vi "Analysis.Result Summaries, Generate Yield Per Day_V3.vi"(8 "LP Yield":dbl[](array[numeric]), 10 "FP Yield":dbl[](array[numeric]), 11 "Dates":timestamp[](array[timestamp])) -> (2 "Yield Per Date":string[][](table), 3 "Yield vs Date":cluster{"Dates":timestamp[], dbl[]}[](graph))   [LabVIEW 2024]
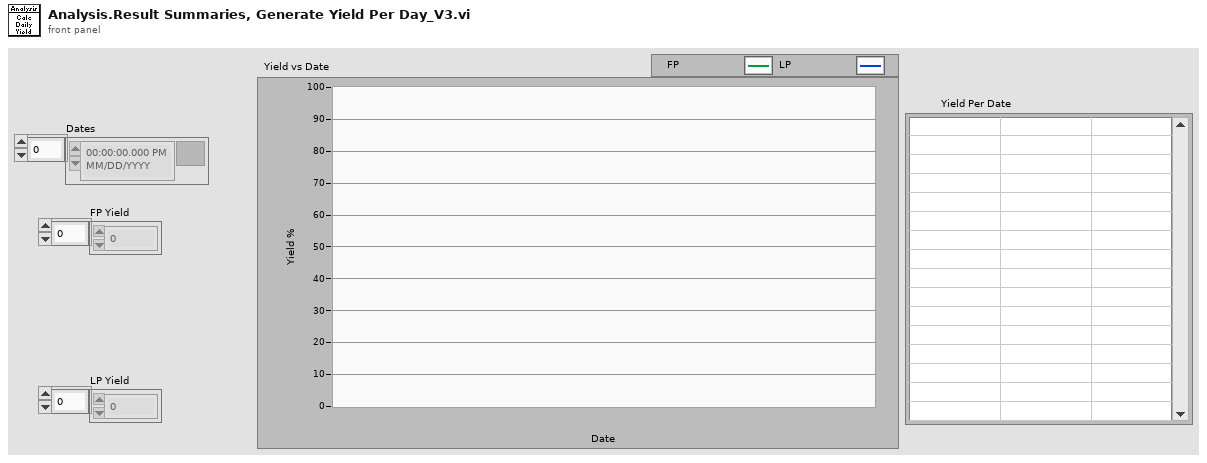
[diagram p1: front panel]
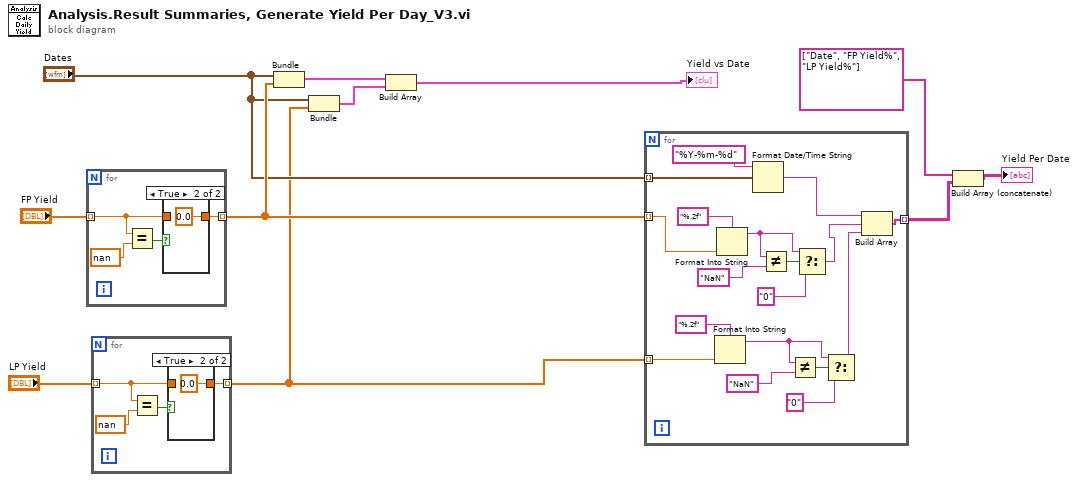
[diagram p0: block diagram]
diagram:
  n1 = for {
    tunnel: "FP Yield" -> [w13] mode=indexing
    tunnel: [w12] -> w7 mode=indexing
    n2 = Equal?(x=w13, y=nan) -> (x = y?=w14:bool)
    n3 = case shown="True" w14 {
      tunnel: w13 -> [w16 _]
      tunnel: [w16 0.0 ("Numeric")] -> w12
      frame False {
      }
      frame True {
      }
    }
  }
  n4 = for {
    tunnel: "LP Yield" -> [w19] mode=indexing
    tunnel: [w18] -> w1 mode=indexing
    n5 = Equal?(x=w19, y=nan) -> (x = y?=w20:bool)
    n6 = case shown="True" w20 {
      tunnel: w19 -> [w22 _]
      tunnel: [w22 0.0 ("Numeric")] -> w18
      frame False {
      }
      frame True {
      }
    }
  }
  n7 = Bundle("Dates"="Dates", w7) -> (w5:cluster{"Dates":timestamp[], dbl[]})  [unwired: 1 in]
  n8 = Bundle("Dates"="Dates", w1) -> (w4:cluster{"Dates":timestamp[], dbl[]})  [unwired: 1 in]
  n9 = Build Array(w5, w4) -> (→"Yield vs Date":cluster{"Dates":timestamp[], dbl[]}[])
  n10 = for {
    tunnel: w7 -> [w39] mode=indexing
    tunnel: "Dates" -> [w41] mode=indexing
    tunnel: [w36] -> w11 mode=indexing
    tunnel: w1 -> [w25] mode=indexing
    n11 = Format Into String(format string="%.2f", w25) -> (resulting string=w29:string)  [unwired: 2 in, 1 out]
    n12 = Format Into String(format string="%.2f", w39) -> (resulting string=w33:string)  [unwired: 2 in, 1 out]
    n13 = Format Date/Time String(time format string (%c)="%Y-%m-%d", seconds (now)=w41) -> (date/time string=w37:string)  [unwired: 1 in]
    n14 = Not Equal?(x=w33, y="NaN") -> (x != y?=w34:bool)
    n15 = Not Equal?(x=w29, y="NaN") -> (x != y?=w28:bool)
    n16 = Select(t=w33, s=w34, f="0") -> (s? t:f=w32:string)
    n17 = Select(t=w29, s=w28, f="0") -> (s? t:f=w24:string)
    n18 = Build Array(w37, w32, w24) -> (w36:string[])
  }
  n19 = Build Array (concatenate)(string[] ["Date", "FP Yield%", "LP Yield%"], w11) -> (→"Yield Per Date":string[][])
